vi "例7.7利用波形图表显示多条曲线.vi"() -> ()   [LabVIEW 2017]
panel:
  out "波形图表 2":T1(graph)
  in  "停止":bool
  out "波形图表":T2(graph)
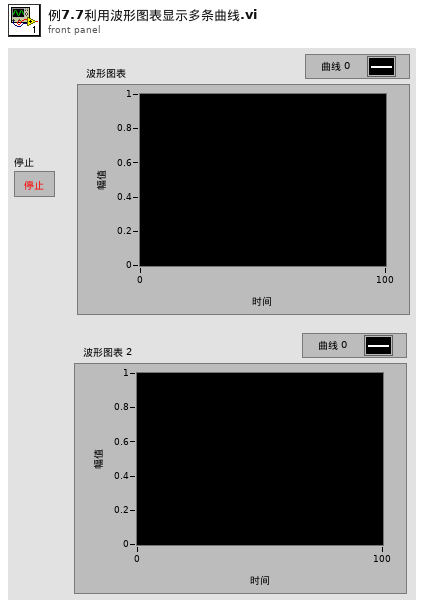
[diagram p1: front panel]
types:
  T1 = cluster{"number: 0 to 1":dbl, "number: 0 to 1":dbl}[]
  T2 = cluster{"number: 0 to 1":dbl, "number: 0 to 1":dbl}
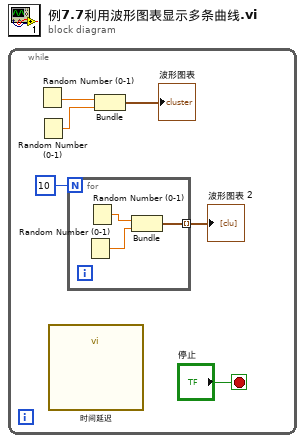
[diagram p0: block diagram]
diagram:
  n1 = while {
    stop <- "停止" stop-if-true
    n2 = Random Number (0-1)() -> (number: 0 to 1=w4:dbl)
    n3 = Random Number (0-1)() -> (number: 0 to 1=w3:dbl)
    n4 = call "时间延迟"() -> ()  [unwired: 11 in, 1 out]
    n5 = for {
      N: 10 -> [_]
      tunnel: [w7] -> w1 mode=indexing
      n6 = Random Number (0-1)() -> (number: 0 to 1=w8:dbl)
      n7 = Random Number (0-1)() -> (number: 0 to 1=w9:dbl)
      n8 = Bundle("number: 0 to 1"=w9, "number: 0 to 1"=w8) -> (w7:T2)  [unwired: 1 in]
    }
    "波形图表 2" <- w1
    n9 = Bundle("number: 0 to 1"=w4, "number: 0 to 1"=w3) -> (→"波形图表":T2)  [unwired: 1 in]
  }
